vi "GetFlags.vi"(8 "error in (no error)":errorcluster, 11 "FlagImpairPluginBase in":refnum<class "FlagImpairPluginBase.lvclass">) -> (0 "error out":errorcluster, 3 "FlagImpairPluginBase out":refnum<class "FlagImpairPluginBase.lvclass">)   [LabVIEW 2017, in "FlagImpairPlugins.lvlib" / "FlagImpairPluginBase.lvclass"]
uses:
  FlagImpairPluginBase.lvclass
  <userlib>/NIST/BaseClasses/Object_class/BaseObject.lvclass
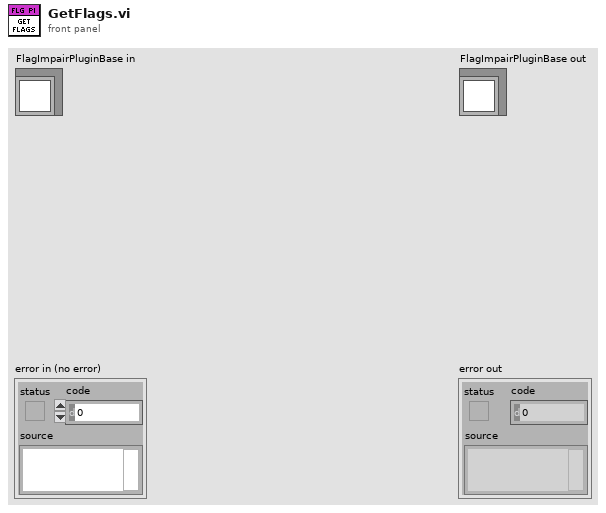
[diagram p1: front panel]
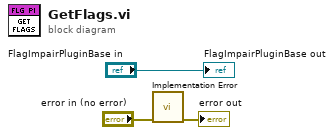
[diagram p0: block diagram]
diagram:
  n1 = call <userlib>:"Implementation Error.vi"("error in (no error)"="error in (no error)") -> ("error out"=→"error out":errorcluster)  [unwired: 10 in]
  "FlagImpairPluginBase out" <- "FlagImpairPluginBase in"
